vi "Voltage - Continuous Output0.vi"(8 "error in (no error)":errorcluster caption="错误输入（无错误）", 10 "波形参数":cluster{"波形类型":u16, "幅值":dbl, "频率":dbl}[](array[cluster])=[{"波形类型"=0, "幅值"=1.0, "频率"=10.0}] {"频率" format="%0.2p"; "幅值" format="%0.2p"; "波形类型" items=["正弦波", "三角波", "方波", "锯齿波"]}, 11 "Hardware Configuration":T2 caption="硬件配置") -> (0 "error out":errorcluster caption="错误输出", 2 "Message":string caption="消息", 3 "Hardware Resources out":T1={"Max Input"=0.0, "Min Input"=0.0, "Sample Rate"=0.0, "Sample Num"=0.0, "DAQmx Task"="", "物理通道"="Dev1/ao0"})   [LabVIEW 2014]
doc: "本范例演示从计算机内存缓冲区连续重新生成数据的方法。\n\n关于引脚和硬件功能的信息，见设备相关的文档。"
uses:
  HardWare/Hardware Configures.ctl
  controls/State.ctl
  support/Message Queue/Enqueue Message (Single).vi
  <vilib>/measure/NI_MABase.lvlib
  <vilib>/DAQmx/configure/timing.llb/DAQmx Timing (Sample Clock).vi
  <vilib>/DAQmx/create/channels.llb/DAQmx Create Channel (AO-Voltage-Basic).vi
  <vilib>/Utility/error.llb/DialogType.ctl
  <vilib>/DAQmx/write.llb/DAQmx Write (Analog 1D Wfm NChan NSamp).vi
  support/Message Queue/Message Queue.lvlib
  HardWare/HardWareConfig.lvlib
panel:
  in  "错误输入（无错误）":errorcluster
  out "错误输出":errorcluster
  in  "停止":bool
  in  "开始":bool
  out "数值":i32
  out "波形图 2":waveform(dbl)[](graph)=[{"t0"=timestamp(0 s since 1904-01-01), "dt"=0.001, "Y"=[]}]
  in  "输出数组":cluster{"波形类型":u16, "幅值":dbl, "频率":dbl}[](array[cluster])=[{"波形类型"=0, "幅值"=1.0, "频率"=10.0}] {"频率" format="%0.2p"; "幅值" format="%0.2p"; "波形类型" items=["正弦波", "三角波", "方波", "锯齿波"]}
  in  "采样数":i32=1000
  in  "停止":bool
  out "波形图":waveform(dbl)[](graph)=[{"t0"=timestamp(0 s since 1904-01-01), "dt"=0.001, "Y"=[]}]
  in  "采样率":dbl=1000.0
  in  "最大电压":dbl=5.0
  in  "最小电压":dbl=-5.0
  in  "物理通道":tag="Dev1/ao0"
  # "触发设置"
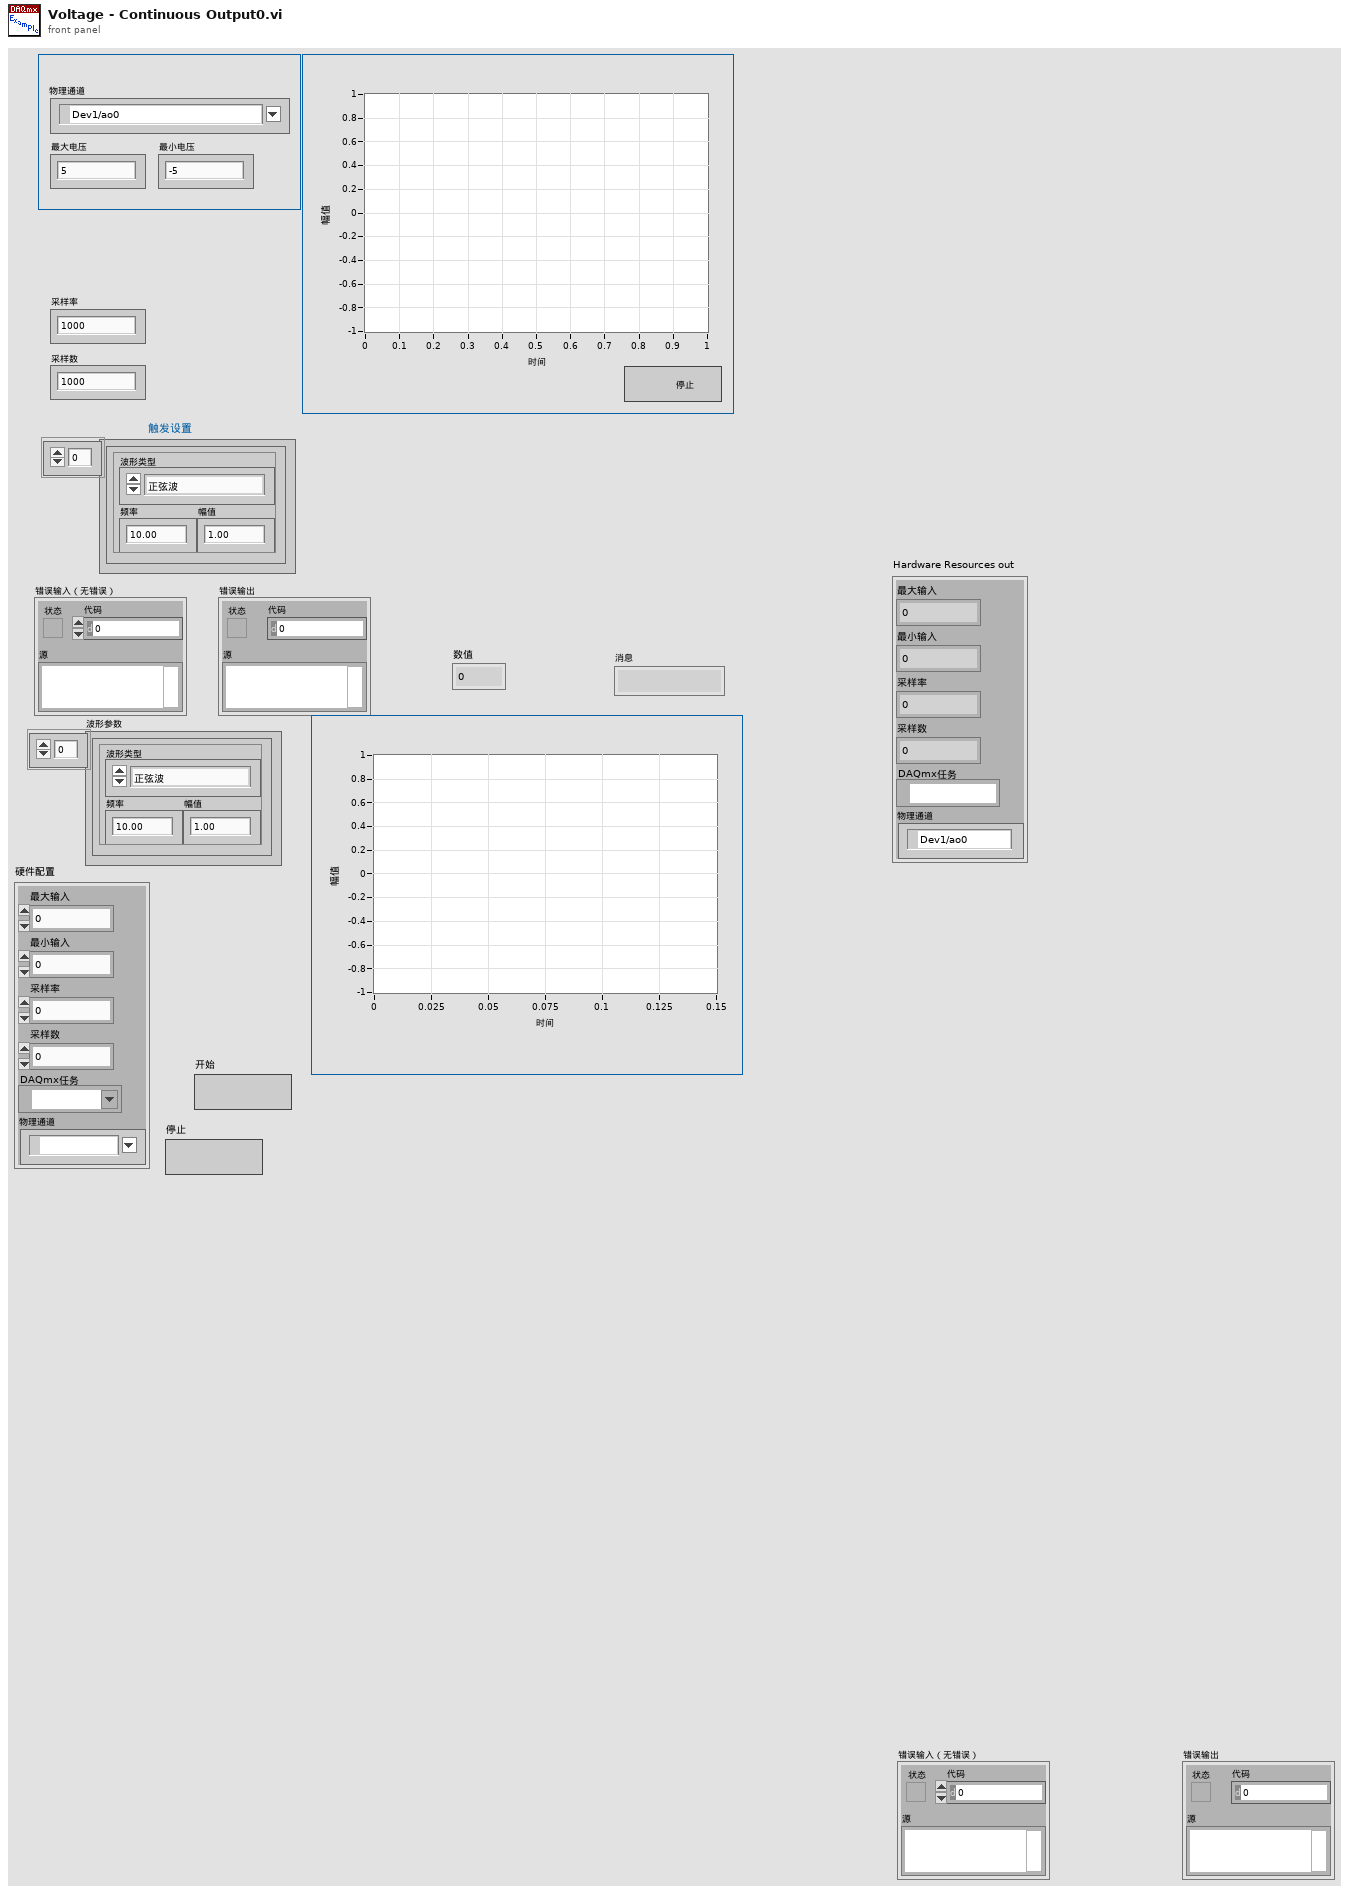
[diagram p1: front panel]
types:
  T1 = typedef "HardWareConfig.lvlib/Hardware Configures.ctl" = cluster{"Max Input":dbl, "Min Input":dbl, "Sample Rate":dbl, "Sample Num":dbl, "DAQmx Task":refnum<k21>, "物理通道":tag}
  T2 = cluster{"Max Input":dbl, "Min Input":dbl, "Sample Rate":dbl, "Sample Num":dbl, "DAQmx Task":refnum<k21>, "物理通道":tag}
  T3 = typedef "Message Queue.lvlib/All Message Queues.ctl" = cluster{"UI":refnum<queue>, "Acquisition":refnum<queue>, "Logging":refnum<queue>}
  T4 = typedef "DialogType.ctl" = u16
  T5 = typedef "State.ctl" = enum16{"Idle", "AOoutputting"}
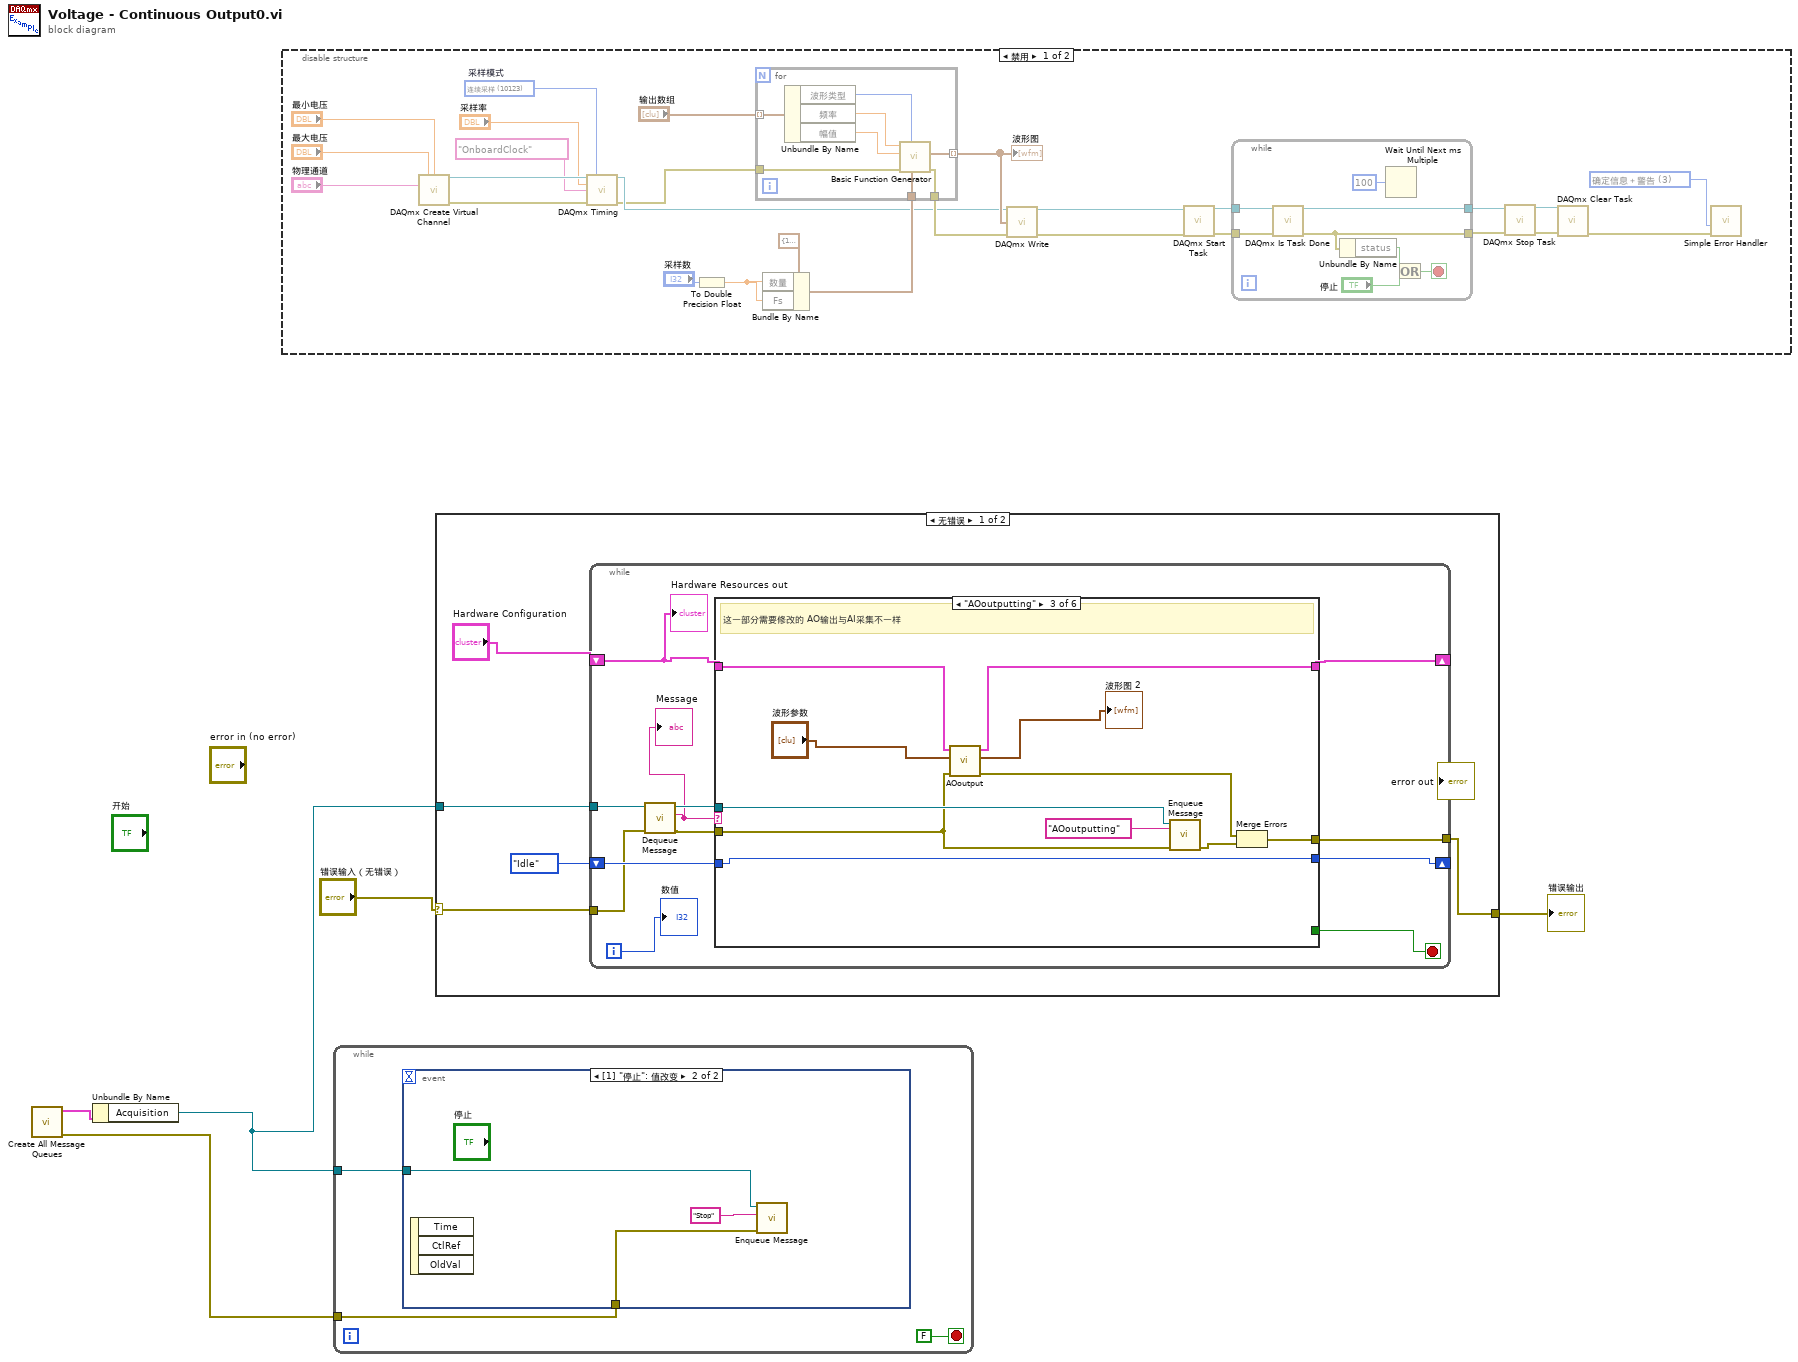
[diagram p0: block diagram]
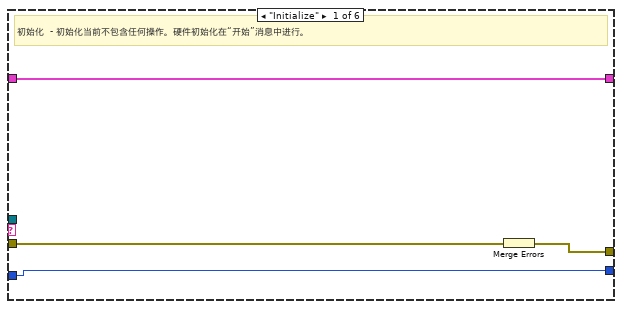
[diagram p2: hidden frame]
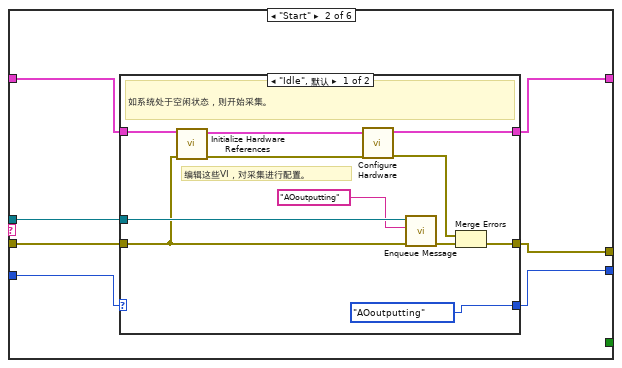
[diagram p3: hidden frame]
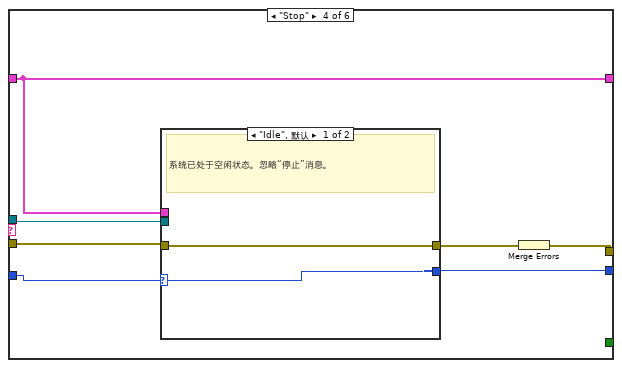
[diagram p5: hidden frame]
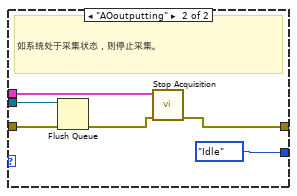
[diagram p6: hidden frame]
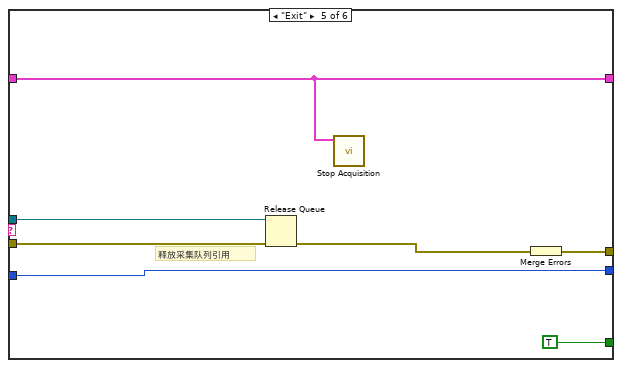
[diagram p7: hidden frame]
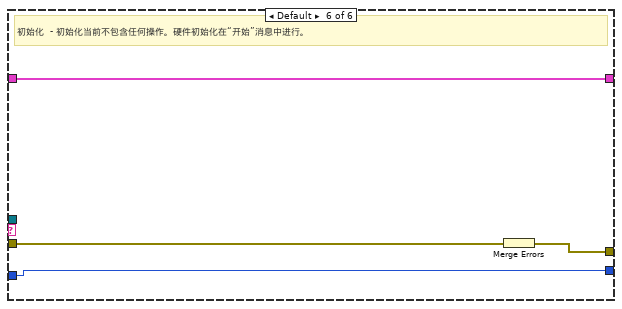
[diagram p8: hidden frame]
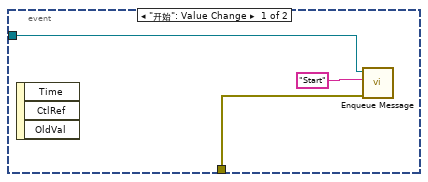
[diagram p10: hidden frame]
diagram:
  n1 = call "Create All Message Queues.vi"() -> ("error out"=w4:errorcluster, "Message Queues out"=w5:T3)  [unwired: 10 in]
  n2 = Unbundle By Name(w5) -> ("Acquisition"=w1:refnum<queue>)
  n3 = disable-structure shown="禁用" {
    frame Disabled {
      w9 = T4 3 items=["无对话框", "确定信息", "继续或停止信息", "确定信息＋警告", "继续/停止＋警告"] ("对话框类型（确定信息：1）")
      w32 = 10123 items=["有限采样"=10178, "连续采样"=10123, "硬件定时单点"=12522]  # 采样模式
      n4 = call-poly <vilib>:"DAQmx Create Virtual Channel.vi"("maximum value"="最大电压", "minimum value"="最小电压", "physical channels"="物理通道") -> ("task out"=w30:refnum<k21>, "error out"=w31:errorcluster)  [unwired: 11 in]
      n5 = call-poly <vilib>:"DAQmx Timing.vi"("task/channels in"=w30, "sample mode"=w32, "rate"="采样率", "source"=tag "OnboardClock" ("采样时钟源"), "error in"=w31) -> ("task out"=w8:refnum<k21>, "error out"=w7:errorcluster)  [unwired: 9 in]
      n6 = To Double Precision Float(number="采样数") -> (double precision float=w6:dbl)
      n7 = Bundle By Name(cluster=cluster{"Fs":dbl, "数量":dbl} {"Fs"=1000.0, "数量"=1000.0} ("采样信息"), "数量"=w6, "Fs"=w6) -> (w20:cluster{"Fs":dbl, "数量":dbl})
      n8 = for {
        tunnel: w20 -> [w40]
        tunnel: [w39] -> w17
        tunnel: "输出数组" -> [w38] mode=indexing
        tunnel: [w34] -> w15 mode=indexing
        tunnel: w7 -> [w33]
        n9 = Unbundle By Name(w38) -> ("波形类型"=w37:u16, "频率"=w36:dbl, "幅值"=w35:dbl)
        n10 = call <vilib>:"Basic Function Generator.vi"("sampling info"=w40, "signal type"=w37, "error in (no error)"=w33, "amplitude"=w35, "frequency"=w36) -> ("error out"=w39:errorcluster, "signal out"=w34:waveform(dbl))  [unwired: 4 in, 1 out]
      }
      "波形图" <- w15
      n11 = call-poly <vilib>:"DAQmx Write.vi"("task/channels in"=w8, "data"=w15, "error in"=w17) -> ("task out"=w19:refnum<k21>, "error out"=w18:errorcluster)  [unwired: 10 in, 1 out]
      n12 = call <vilib>:"DAQmx Start Task.vi"("task/channels in"=w19, "error in"=w18) -> ("task out"=w29:refnum<k21>, "error out"=w28:errorcluster)  [unwired: 12 in]
      n13 = while {
        tunnel: w29 -> [w48]
        tunnel: w28 -> [w47]
        tunnel: [w44] -> w10
        tunnel: [w45] -> w11
        stop <- w46 stop-if-true
        n14 = call <vilib>:"DAQmx Is Task Done.vi"("task/channels in"=w48, "error in"=w47) -> ("task out"=w45:refnum<k21>, "error out"=w44:errorcluster)  [unwired: 11 in, 1 out]
        n15 = Unbundle By Name(w44) -> ("status"=w43:bool)
        n16 = Wait Until Next ms Multiple(millisecond multiple=u32 100 ("毫秒倍数")) -> ()  [unwired: 1 out]
        n17 = Or(x=w43, y="停止") -> (x .or. y?=w46:bool)
      }
      n18 = call <vilib>:"DAQmx Stop Task.vi"("task/channels in"=w11, "error in"=w10) -> ("task out"=w13:refnum<k21>, "error out"=w12:errorcluster)  [unwired: 12 in]
      n19 = call <vilib>:"DAQmx Clear Task.vi"("task in"=w13, "error in"=w12) -> ("error out"=w27:errorcluster)  [unwired: 13 in]
      n20 = call <vilib>:"Simple Error Handler.vi"("type of dialog (OK msg:1)"=w9, "error in (no error)"=w27) -> ()  [unwired: 3 in, 5 out]
    }
    frame Enabled {
    }
  }
  n21 = while {
    tunnel: w1 -> [w50]
    tunnel: w4 -> [w49]
    stop <- FALSE stop-if-true
    n22 = event shown="[1] \"停止\": 值改变" {
      selector: _ -> [_ _]
      dyn-events: _ -> [_ _]
      timeout: _ -> [_ _]
      tunnel: w50 -> [w53 w56]
      tunnel: w49 -> [w52 w55]
      event "开始": Value Change {
        n23 = event-data() -> ()  [unwired: 1 in, 3 out]
        n24 = call-poly "Enqueue Message.vi"("error in (no error)"=w52, "Message"="Start", "Message Queue"=w53) -> ()  [unwired: 7 in, 2 out]
      }
      event "停止": Value Change {
        n25 = event-data() -> ()  [unwired: 1 in, 3 out]
        n26 = call-poly "Enqueue Message.vi"("error in (no error)"=w55, "Message"="Stop", "Message Queue"=w56) -> ()  [unwired: 7 in, 2 out]
      }
    }
  }
  n27 = case shown="无错误" "错误输入（无错误）" {
    selector: "错误输入（无错误）" -> [w61 w137]
    tunnel: [w62 w137] -> w3
    tunnel: w1 -> [w59 _]
    frame No Error {
      n28 = while {
        tunnel: [w74] -> w62
        tunnel: w61 -> [w67]
        shift-right: [w72] -> _
        shift-left: State."Idle" ("State") -> [w71]
        shift-right: [w73] -> _
        shift-left: "Hardware Configuration" -> [w65]
        tunnel: w59 -> [w66]
        i -> [w63]
        stop <- w70 stop-if-true
        n29 = call "Dequeue Message.vi"("error in (no error)"=w67, "Message Queue"=w66) -> ("error out"=w68:errorcluster, "Message"=w64:string, "dup Message Queue"=w69:refnum<queue>)  [unwired: 6 in, 1 out]
        "Message" <- w64
        n30 = case shown="\"AOoutputting\"" w64 {
          tunnel: [w76 w80 w107 w113 w128 w134] -> w74
          tunnel: w65 -> [w78 w81 w110 w111 w126 w136]
          tunnel: [w78 w79 w109 w111 w126 w136] -> w73
          tunnel: w68 -> [w77 w83 w104 w117 w131 w135]
          tunnel: [w75 w84 w102 w114 w130 w133] -> w72
          tunnel: w71 -> [w75 w85 w102 w115 w130 w133]
          tunnel: w69 -> [_ w82 w105 w116 w132 _]
          tunnel: [_ _ _ _ TRUE _] -> w70
          frame "Initialize" {
            # "初始化  - 初始化当前不包含任何操作。硬件初始化在“开始”消息中进行。"
            n31 = Merge Errors(w77) -> (w76:errorcluster)
          }
          frame "Start" {
            n32 = case shown="\"Idle\", 默认" w85 {
              selector: w85 -> [_ w97]
              tunnel: [w96 w99] -> w80
              tunnel: w81 -> [w90 w98]
              tunnel: w83 -> [w89 w99]
              tunnel: w82 -> [w94 _]
              tunnel: [w86 w98] -> w79
              tunnel: [State."AOoutputting" ("State") w97] -> w84
              frame "Idle", Default {
                # "编辑这些VI，对采集进行配置。"
                # "如系统处于空闲状态，则开始采集。"
                n33 = call "Initialize Hardware References.vi"("error in (no error)"=w89, "Hardware Resources in"=w90) -> ("error out"=w88:errorcluster, "Hardware Resources out"=w87:T1)  [unwired: 8 in]
                n34 = call "Configure Hardware.vi"("error in (no error)"=w88, "Hardware Resources in"=w87) -> ("error out"=w93:errorcluster, "Hardware Resources out"=w86:T1)  [unwired: 8 in]
                n35 = call-poly "Enqueue Message.vi"("error in (no error)"=w89, "Message"="AOoutputting", "Message Queue"=w94) -> ("error out"=w95:errorcluster)  [unwired: 7 in, 1 out]
                n36 = Merge Errors(w93, w95) -> (w96:errorcluster)
              }
              frame "AOoutputting" {
                # "系统已开始采集。忽略“开始”消息。"
              }
            }
          }
          frame "AOoutputting" {
            # "这一部分需要修改的 AO输出与AI采集不一样"
            n37 = call "AOoutput.vi"("error in (no error)"=w104, "波形参数"="波形参数", "Hardware Resources in"=w110) -> ("error out"=w108:errorcluster, "波形图"=→"波形图 2":waveform(dbl)[], "Hardware Resources out"=w109:T1)  [unwired: 6 in]
            n38 = call-poly "Enqueue Message.vi"("error in (no error)"=w104, "Message"="AOoutputting", "Message Queue"=w105) -> ("error out"=w103:errorcluster)  [unwired: 7 in, 1 out]
            n39 = Merge Errors(w108, w103) -> (w107:errorcluster)
          }
          frame "Stop" {
            n40 = case shown="\"Idle\", 默认" w115 {
              selector: w115 -> [w119 _]
              tunnel: w117 -> [w118 w125]
              tunnel: w116 -> [_ w124]
              tunnel: [w119 State."Idle" ("State")] -> w114
              tunnel: [w118 w120] -> w112
              tunnel: w111 -> [_ w122]
              frame "Idle", Default {
                # "系统已处于空闲状态。忽略“停止”消息。"
              }
              frame "AOoutputting" {
                # "如系统处于采集状态，则停止采集。"
                n41 = Flush Queue(queue=w124, error in (no error)=w125) -> (error out=w121:errorcluster)  [unwired: 2 out]
                n42 = call "Stop Acquisition.vi"("error in (no error)"=w121, "Hardware Resources in"=w122) -> ("error out"=w120:errorcluster)  [unwired: 9 in]
              }
            }
            n43 = Merge Errors(w112) -> (w113:errorcluster)
          }
          frame "Exit" {
            # "释放采集队列引用"
            n44 = Release Queue(queue=w132, error in (no error)=w131) -> (error out=w127:errorcluster)  [unwired: 1 in, 2 out]
            n45 = call "Stop Acquisition.vi"("Hardware Resources in"=w126) -> ()  [unwired: 10 in, 1 out]
            n46 = Merge Errors(w127) -> (w128:errorcluster)
          }
          frame Default {
            # "初始化  - 初始化当前不包含任何操作。硬件初始化在“开始”消息中进行。"
            n47 = Merge Errors(w135) -> (w134:errorcluster)
          }
        }
        "Hardware Resources out" <- w65
        "数值" <- w63
      }
    }
    frame Error {
    }
  }
  "错误输出" <- w3
